vi "FTW-JSON-Object-GetElement-String.vi"(0 "JSON Object":refnum<class "FTW-JSON.lvclass">, 5 "Key":string, 11 "error in":errorcluster) -> (4 "JSON Object out":refnum<class "FTW-JSON.lvclass">, 6 "Value":string, 8 "Found?":bool, 15 "error out":errorcluster)   [LabVIEW 2013, in "FTW-JSON.lvclass"]
uses:
  FTW-JSON.lvclass
  FTW-JSON.lvclass/FTW-JSON.ctl
panel:
  # "Inputs"
  # "Outputs"
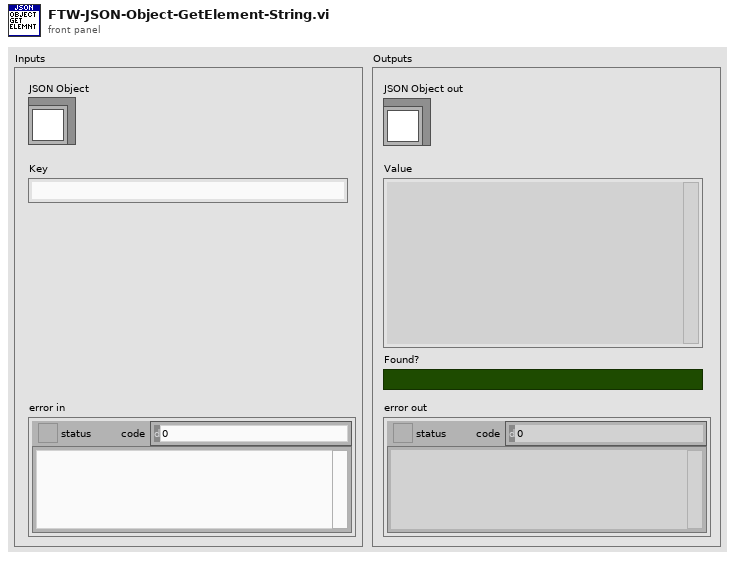
[diagram p1: front panel]
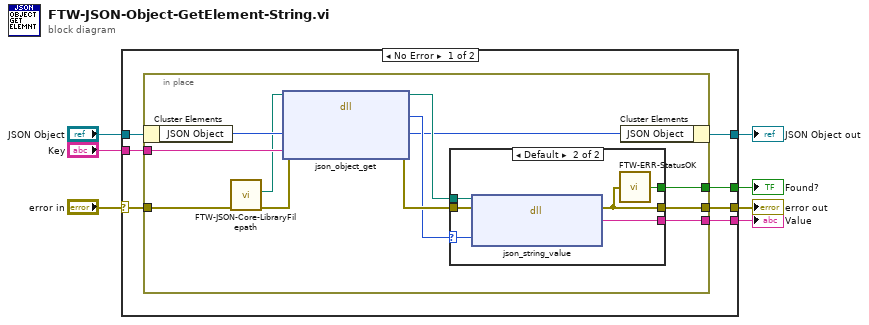
[diagram p0: block diagram]
diagram:
  n1 = case shown="No Error" "error in" {
    selector: "error in" -> [w14 w35]
    tunnel: [w10 w35] -> w7
    tunnel: [w12 w34] -> w5
    tunnel: "JSON Object" -> [w13 w34]
    tunnel: "Key" -> [w11 _]
    tunnel: [w9 _] -> w2
    tunnel: [w8 _] -> w1
    frame No Error {
      n2 = in-place {
        in-place-border: w14 -> [w26]
        in-place-border: w11 -> [w24]
        in-place-border: [w20] -> w10
        in-place-border: [w19] -> w9
        in-place-border: [w15] -> w8
        n3 = in-place-cluster #1(w13) -> ("JSON Object"=w25:i64)
        n4 = call "FTW-JSON-Core-LibraryFilepath.vi"("error in"=w26) -> ("error out"=w23:errorcluster, "JSON Library Filepath"=w22:path)  [unwired: 9 in]
        n5 = dll-call lib="?" fn="json_object_get"(path in=w22, error in=w23, "JSON Object Pointer"=w25, "Element Key"=w24) -> (path out=w18:path, error out=w21:errorcluster, "JSON Element Pointer"=w17:i64, "JSON Object Pointer"=w16:i64)  [unwired: 2 in]
        n6 = case shown="Default" w17 {
          selector: w17 -> [_ w30]
          tunnel: w21 -> [w27 w33]
          tunnel: [w27 w29] -> w20
          tunnel: [_ w32] -> w19
          tunnel: w18 -> [_ w31]
          tunnel: [_ w28] -> w15
          frame 0 {
          }
          frame Default {
            n7 = dll-call lib="?" fn="json_string_value"(path in=w31, error in=w33, "JSON Element Pointer"=w30) -> (error out=w29:errorcluster, "String Value"=w32:string)  [unwired: 2 in, 1 out]
            n8 = call "FTW-ERR-StatusOK.vi"("error to check"=w29) -> ("Status OK?"=w28:bool)
          }
        }
        n9 = in-place-cluster #1("JSON Object"=w16) -> (w12:refnum<class "FTW-JSON.lvclass">)
      }
    }
    frame Error {
    }
  }
  "error out" <- w7
  "JSON Object out" <- w5
  "Value" <- w2
  "Found?" <- w1
